vi "Destroy.vi"(8 "error in (no error)":errorcluster, 11 "Apriltag Detector in":refnum<class "AprilTag Detector.lvclass">) -> (0 "error out":errorcluster)   [LabVIEW 2020, in "feature_detection.lvlib" / "AprilTag Detector.lvclass"]
doc: "Destroy the detector."
uses:
  AprilTag Detector.lvclass
  AprilTag Detector.lvclass/AprilTag Detector.ctl
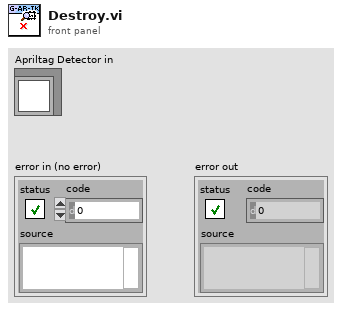
[diagram p1: front panel]
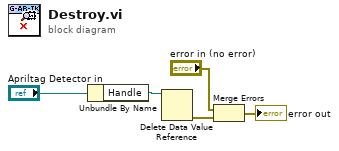
[diagram p0: block diagram]
diagram:
  n1 = Unbundle By Name("Apriltag Detector in") -> ("Handle"=w4:refnum<data-value>)
  n2 = Delete Data Value Reference(data value reference=w4) -> (error out=w2:errorcluster)  [unwired: 1 in, 1 out]
  n3 = Merge Errors("error in (no error)", w2) -> (→"error out":errorcluster)
